vi "OAT Sampled Power Spectrum (Single Channel).vi"(6 "window info":T4={"window type"=10, "window length"=2048} {"window type" items=["None"=0, "Hanning"=1, "Hamming"=2, "Blackman-Harris"=3, "Exact Blackman"=4, "Blackman"=5, "Flat Top"=6, "4 Term B-Harris"=7, "7 Term B-Harris"=8, "Low Sidelobe"=9, "Gaussian"=62]; "window length" min=0}, 7 "dB On (T)":bool=TRUE, 8 "error in (no error)":errorcluster, 10 "channel info":T1={"sensor sensitivity"=1000.0, "engineering units"=1, "dB reference"=1.0, "custom label"="EU", "weighting filter"=0, "pregain"=0.0} {"pregain" format="%.2f"; "weighting filter" items=["Linear", "A-weighting", "B-weighting", "C-weighting", "ITU-R 468-4", "Dolby", "CCITT", "C-message", "Wb", "Wc", "Wd", "We", "Wf", "Wh", "Wj", "Wk", "Wm", "AES17 20 kHz lowpass", "AES17 40 kHz lowpass", "AES17 20 kHz highpass", "AES17 40 kHz highpass"]; "dB reference" format="%^.1e"; "engineering units" items=["custom..."=0, "V"=1, "A"=21, "C"=30, "pC"=31, "s"=32, "-"=29, "Pa"=2, "N"=20, "g"=3, "m/s^2"=4, "m/s"=5, "m"=6, "mm/s"=12, "mm"=13, "micron/s"=14, "micron"=15, "in/s^2"=7, "in/s"=8, "in"=9, "mil/s"=10, "mil"=11, "rad/s^2"=16, "rad/s"=17, "rad"=18, "deg/s^2"=26, "deg/s"=27, "deg"=28, "RPM"=22, "cycle/s^2"=23, "Hz"=24, "cycle"=25, "strain"=19]; "sensor sensitivity" format="%#_5f"}, 11 "resampled signal":cluster{"r0":dbl, "dr":dbl, "Y":dbl[]}={"r0"=0.0, "dr"=1.0, "Y"=[]} {"r0" format="%.2p"; "dr" format="%.2p"; "Y" format="%.2f"}) -> (0 "error out":errorcluster, 2 "unit label":string, 3 "order spectrum":T5={"order 0"=0.0, "delta order"=1.0, "magnitude"=[]} {"order 0" format="%.2p"; "delta order" format="%.2p"; "magnitude" format="%.2f"})   [LabVIEW 2017]
doc: "Computes the single-sided, scaled auto power spectrum of a time-domain signal. You can define the number of frequency bins."
uses:
  <vilib>/addons/Sound and Vibration/Order Analysis/Ref Gabor Order Tracking/window information.ctl
  <vilib>/addons/_NISVFA/_Shared subVIs/Controls/svc_Channel Info.ctl
  <vilib>/addons/_NISVFA/_Shared subVIs/Controls/svc_Engineering Units Text Ring.ctl
  <vilib>/addons/_NISVFA/_Shared subVIs/Controls/svc_Weighting Filter Text Ring.ctl
  <vilib>/addons/Sound and Vibration/Order Analysis/Resample Order Tracking/SubVIs/OAT Verify Resampled Signal (Single Channel).vi
  <vilib>/Analysis/NI_AALPro.lvlib
  <vilib>/addons/Sound and Vibration/Order Analysis/Resample Order Tracking/SoundVib_Resampling.lvlib
  <vilib>/addons/Sound and Vibration/Order Analysis/Gabor Order Tracking/SoundVib_Gabor.lvlib
panel:
  # "OAT Sampled Power Spectrum (Single Channel)"
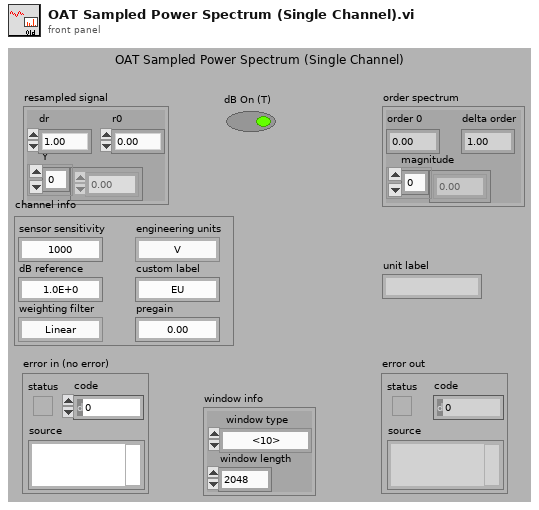
[diagram p1: front panel]
types:
  T1 = typedef "svc_Channel Info.ctl" = cluster{"sensor sensitivity":dbl, "engineering units":T2, "dB reference":dbl, "custom label":string, "weighting filter":T3, "pregain":dbl}
  T2 = typedef "svc_Engineering Units Text Ring.ctl" = u16
  T3 = typedef "svc_Weighting Filter Text Ring.ctl" = u16
  T4 = typedef "SoundVib_Gabor.lvlib/window information.ctl" = cluster{"window type":u32, "window length":i32}
  T5 = cluster{"order 0":dbl, "delta order":dbl, "magnitude":dbl[]}
  T6 = cluster{"df":dbl, "df":dbl, "log view [dB EU]":dbl[]}
  T7 = cluster{"df":dbl, "df":dbl, "log view scaled signal":dbl[]}
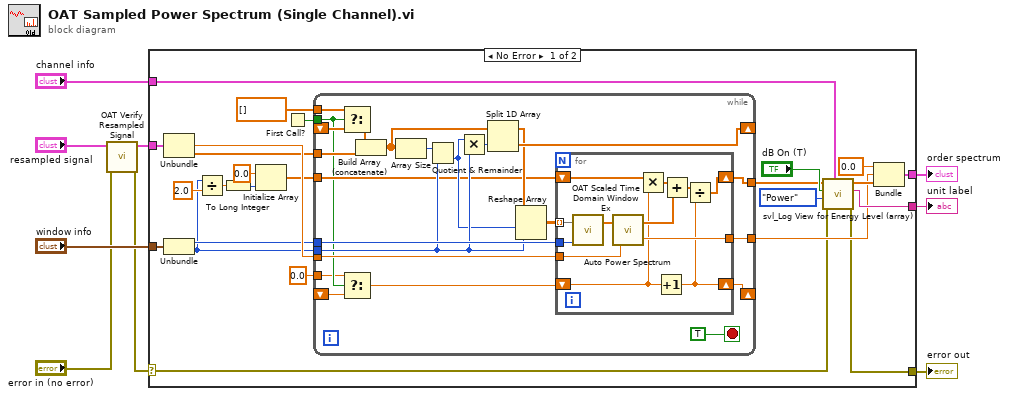
[diagram p0: block diagram]
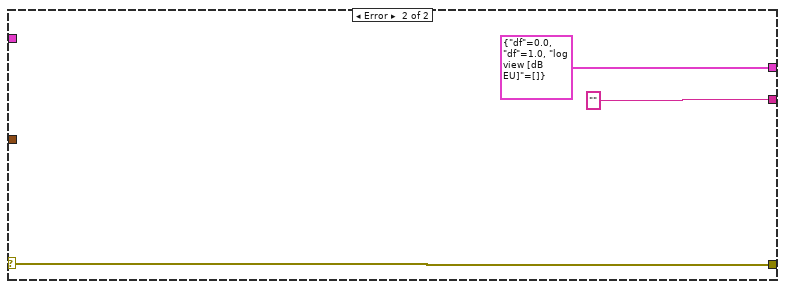
[diagram p2: hidden frame]
diagram:
  n1 = call-poly <vilib>:"OAT Verify Resampled Signal.vi"("error in (no error)"="error in (no error)", "resampled signal"="resampled signal") -> ("error out"=w4:errorcluster, "resampled signal dup"=w2:cluster{"r0":dbl, "dr":dbl, "Y":dbl[]})  [unwired: 7 in, 1 out]
  n2 = case shown="No Error" w4 {
    selector: w4 -> [w23 w70]
    tunnel: "window info" -> [w34 _]
    tunnel: w2 -> [w33 _]
    tunnel: [w29 "" ("unit label")] -> w8
    tunnel: [w25 T6 {"df"=0.0, "df"=1.0, "log view [dB EU]"=[]}] -> w7
    tunnel: "channel info" -> [w24 _]
    tunnel: [w22 w70] -> w1
    frame No Error {
      n3 = Unbundle(w33) -> ("dr"=w32:dbl, "Y"=w20:dbl[])  [unwired: 1 out]
      n4 = Unbundle(w34) -> ("window type"=w19:u32, "window length"=w14:i32)
      n5 = Divide(x=w14, y=2.0) -> (x/y=w16:dbl)
      n6 = To Long Integer(number=w16) -> (32bit integer=w17:i32)
      n7 = Initialize Array(0.0 ("element"), w17) -> (w12:dbl[])
      n8 = First Call?() -> (First Call?: T/F=w13:bool)
      n9 = while {
        tunnel: w32 -> [w56]
        tunnel: [w55] -> w27
        tunnel: [w41] -> w21
        tunnel: w14 -> [w44]
        tunnel: w20 -> [w51]
        tunnel: w19 -> [w53]
        shift-right: [w48] -> _
        shift-left: _ -> [w46]
        tunnel: w13 -> [w40]
        tunnel: w12 -> [w42]
        shift-right: [w37] -> _
        shift-left: _ -> [w36]
        tunnel: 0.0 ("t") -> [w39]
        tunnel: dbl[] [] ("Y") -> [w35]
        stop <- TRUE stop-if-true
        n10 = Select(t=w35, s=w40, f=w46) -> (s? t:f=w45:dbl[])
        n11 = Select(t=w39, s=w40, f=w36) -> (s? t:f=w38:dbl)
        n12 = Build Array (concatenate)(w45, w51) -> (w50:dbl[])
        n13 = Array Size(array=w50) -> (size(s)=w57:i32)
        n14 = Quotient & Remainder(x=w57, y=w44) -> (floor(x/y)=w43:i32)  [unwired: 1 out]
        n15 = Multiply(x=w43, y=w44) -> (x*y=w49:i32)
        n16 = Split 1D Array(array=w50, index=w49) -> (first subarray=w47:dbl[], second subarray=w48:dbl[])
        n17 = Reshape Array(w47, w43, w44) -> (w54:dbl[][])
        n18 = for {
          tunnel: w56 -> [w65]
          tunnel: [w69] -> w55
          shift-right: [w60] -> w41
          shift-left: w42 -> [w62]
          tunnel: w54 -> [w67] mode=indexing
          tunnel: w53 -> [w64]
          shift-right: [w58] -> w37
          shift-left: w38 -> [w59]
          n19 = call <vilib>:"OAT Scaled Time Domain Window Ex.vi"("window type"=w64, "X"=w67) -> ("y"=w66:dbl[])  [unwired: 1 out]
          n20 = call <vilib>:"Auto Power Spectrum.vi"("dt"=w65, "Signal (V)"=w66) -> ("df"=w69:dbl, "Power Spectrum (V^2 rms)"=w68:dbl[])
          n21 = Multiply(x=w62, y=w59) -> (x*y=w63:dbl[])
          n22 = Increment(x=w59) -> (x+1=w58:dbl)
          n23 = Add(x=w63, y=w68) -> (x+y=w61:dbl[])
          n24 = Divide(x=w61, y=w58) -> (x/y=w60:dbl[])
        }
      }
      n25 = call <vilib>:"svl_Log View for Energy Level (array).vi"("channel info"=w24, "error in (no error)"=w23, "view mode"=enum16{"Power", "Amplitude"}."Power", "dB On (T)"="dB On (T)", "scaled signal"=w21) -> ("error out"=w22:errorcluster, "unit label"=w29:string, "log view scaled signal"=w28:dbl[])  [unwired: 4 in]
      n26 = Bundle("df"=0.0, "df"=w27, "log view scaled signal"=w28) -> (w25:T7)  [unwired: 1 in]
    }
    frame Error {
    }
  }
  "order spectrum" <- w7
  "unit label" <- w8
  "error out" <- w1
